vi "Parse Offsets.vi"(9 "Line":string, 11 "LBCB Selected":T1) -> ()   [LabVIEW 2009]
uses:
  Data Access Objects/Metadata/LBCB Number.ctl
  Cartesian Measurment Actions.ctl
  Cartesian Data type.ctl
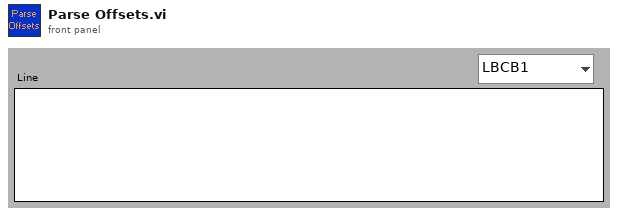
[diagram p1: front panel]
types:
  T1 = typedef "LBCB Number.ctl" = enum16{"LBCB1", "LBCB2"}
  T2 = typedef "Cartesian Data type.ctl" = cluster{"Displacements":dbl[], "Forces":dbl[], "Displacement Commands":dbl[]}
  T3 = typedef "Cartesian Measurment Actions.ctl" = enum16{"Set Data", "Get", "Init", "Set Offsets"}
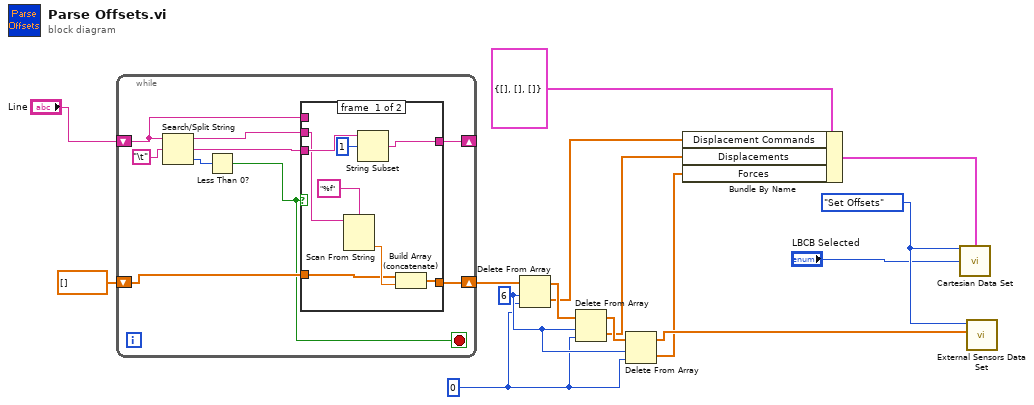
[diagram p0: block diagram]
diagram:
  w1 = 0 ("index")
  w9 = 6 ("length")
  w13 = Cartesian_Measurment_Actions."Set Offsets" ("Measurement Actions")
  n1 = while {
    shift-right: [w21] -> _
    shift-left: "Line" -> [w16]
    shift-right: [w19] -> w12
    shift-left: dbl[] [] -> [w18]
    stop <- w17 stop-if-true
    n2 = Search/Split String(string=w16, search string/char (-)="\t") -> (substring before match=w20:string, match + rest of string=w22:string, offset of match=w24:i32)  [unwired: 1 in]
    n3 = Less Than 0?(x=w24) -> (x < 0?=w17:bool)
    n4 = case shown="False" w17 {
      tunnel: w22 -> [w32 _]
      tunnel: [w30 w33] -> w21
      tunnel: w20 -> [w29 _]
      tunnel: [w26 w34] -> w19
      tunnel: w18 -> [w25 w34]
      tunnel: w16 -> [_ w33]
      frame #0 {
        n5 = Scan From String(format string="%f", input string=w29) -> (output 1=w27:dbl)  [unwired: 3 in, 3 out]
        n6 = String Subset(string=w32, offset (0)=1) -> (substring=w30:string)  [unwired: 1 in]
        n7 = Build Array (concatenate)(w25, w27) -> (w26:dbl[])
      }
      frame #1 {
      }
    }
  }
  n8 = Delete From Array(array=w12, length=w9, index=w1) -> (deleted portion=w7:dbl[], array with subset deleted=w8:dbl[])
  n9 = Delete From Array(array=w8, length=w9, index=w1) -> (deleted portion=w5:dbl[], array with subset deleted=w6:dbl[])
  n10 = Delete From Array(array=w6, length=w9, index=w1) -> (deleted portion=w3:dbl[], array with subset deleted=w4:dbl[])
  n11 = Bundle By Name(cluster=T2 {"Displacements"=[], "Forces"=[], "Displacement Commands"=[]} ("Cartesian Offsets In"), "Displacement Commands"=w7, "Displacements"=w5, "Forces"=w3) -> (w10:T2)
  n12 = call "Cartesian Data Set.vi"("Measurement Actions"=w13, "Cartesian Offsets In"=w10, "LBCB Selected"="LBCB Selected") -> ()  [unwired: 9 in, 4 out]
  n13 = call "External Sensors Data Set.vi"("Input Data"=w4, "Measurement Actions"=w13) -> ()  [unwired: 6 in, 4 out]
